vi "IVI DC Power Supply RT Driver VI.vi"(6 "Device Clock":string, 9 "Device Inputs FIFO":refnum<k33>, 10 "Device Outputs FIFO":refnum<k33>, 11 "Device Reference":T1 format="%.0x") -> ()   [LabVIEW 2011, in "IVI DC Power Supply Custom Device.lvlib"]
uses:
  IVI DC Power Supply Custom Device.lvlib
  <vilib>/NI Veristand/Custom Device API/Custom Device Item Ref.ctl
  <vilib>/NI Veristand/Custom Device API/Custom Device Channel Type.ctl
  <vilib>/Platform/TimedLoop/XDataNode/timing_clust.ctl
  <vilib>/Platform/TimedLoop/XDataNode/nitl_modes.ctl
  <vilib>/Platform/TimedLoop/XDataNode/wakeup.ctl
  Global.vi
  <vilib>/NI Veristand/Custom Device API/Get Item Property (Double).vi
  <vilib>/Platform/TimedLoop/XDataNode/XDataNode.xnode
  <vilib>/Platform/TimedLoop/XDataNode/XDNodeRunTimeDep.lvlib
  <vilib>/NI Veristand/Custom Device API/Custom Device API.lvlib
  <vilib>/NI Veristand/Custom Device Tools/Custom Device Utility Library/Custom Device Utility Library.lvlib
panel:
  in  "Status Notifier":refnum<notifier>
  # "Custom Device Template\nv1.0"
  # "Use this template as a starting point for creating a custom device code module. The input controls shown here are specially named controls that the system will use to provide the device loop with data. The controls are not required for the device loop to run. For instance, if the device doesn't produce any output data, then you don't need the Device Outputs FIFO control. If you do use these controls, however, they need to have these exact names to be functional."
  # "The optional status notifier element is used to notify the RT engine of the last state of the custom device, and to indicate the device has completed execution. If this control is not used, a default No Error value is returned to the system when the device finishes execution.\n\nNote: This error state is not checked until the system shuts down. Use an output status channel to send more immediate status values to the system."
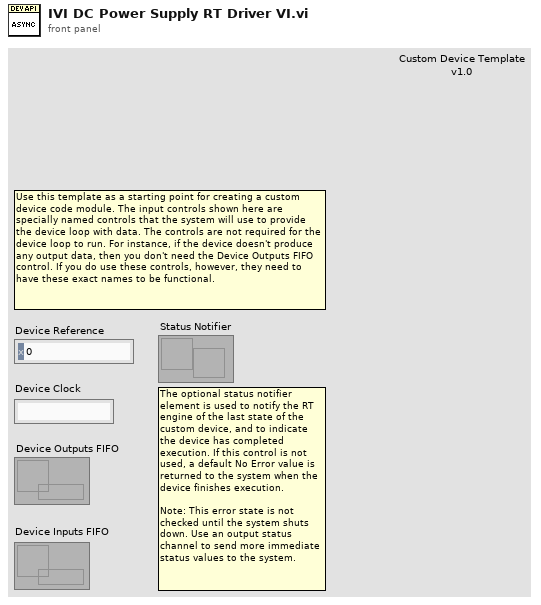
[diagram p1: front panel]
types:
  T1 = typedef "Custom Device API.lvlib/Custom Device Item Ref.ctl" = u64
  T2 = typedef "Custom Device API.lvlib/Custom Device Channel Type.ctl" = enum16{"Input", "Output"}
  T3 = typedef "Custom Device API.lvlib/Custom Device Timed Loop Priority.ctl" = enum32{"Low", "Medium", "High"}
  T4 = typedef "XDNodeRunTimeDep.lvlib/timing_clust.ctl" = cluster{"Expected End [f-1]":u64, "Actual End [f-1]":u64, "Finished Late? [f-1]":bool, "Expected End [i-1]":u64, "Actual End [i-1]":u64, "Finished Late? [i-1]":bool, "Expected Start [i]":u64, "Actual Start [i]":u64, "Expected Start [f]":u64, "Actual Start [f]":u64, "Source Name":string, "Structure Name":string, "Period":i64, "Deadline":i64, "Offset":i64, "Start":i64, "Priority":i32, "Timeout":i32, "Mode":T5, "Wakeup Reason":T6, "Error":errorcluster, "Source Type":string, "Secondary Source Type":string, "Global End Time":u64, "Global Start Time":u64, "Frame Duration":u64, "Iteration Duration":u64, "Assigned CPU":i32, "I/O Scan Engine Mode":u32}
  T5 = typedef "XDNodeRunTimeDep.lvlib/nitl_modes.ctl" = enum32{"No Change", "Process missed periods, maintain original phase", "Discard missed periods, maintain original phase", "Process missed periods, ignore original phase", "Discard missed periods, ignore original phase"}
  T6 = typedef "XDNodeRunTimeDep.lvlib/wakeup.ctl" = enum32{"Normal", "Aborted", "Asynchronous wakeup", "Timing source error", "Timed loop error", "Timeout"}
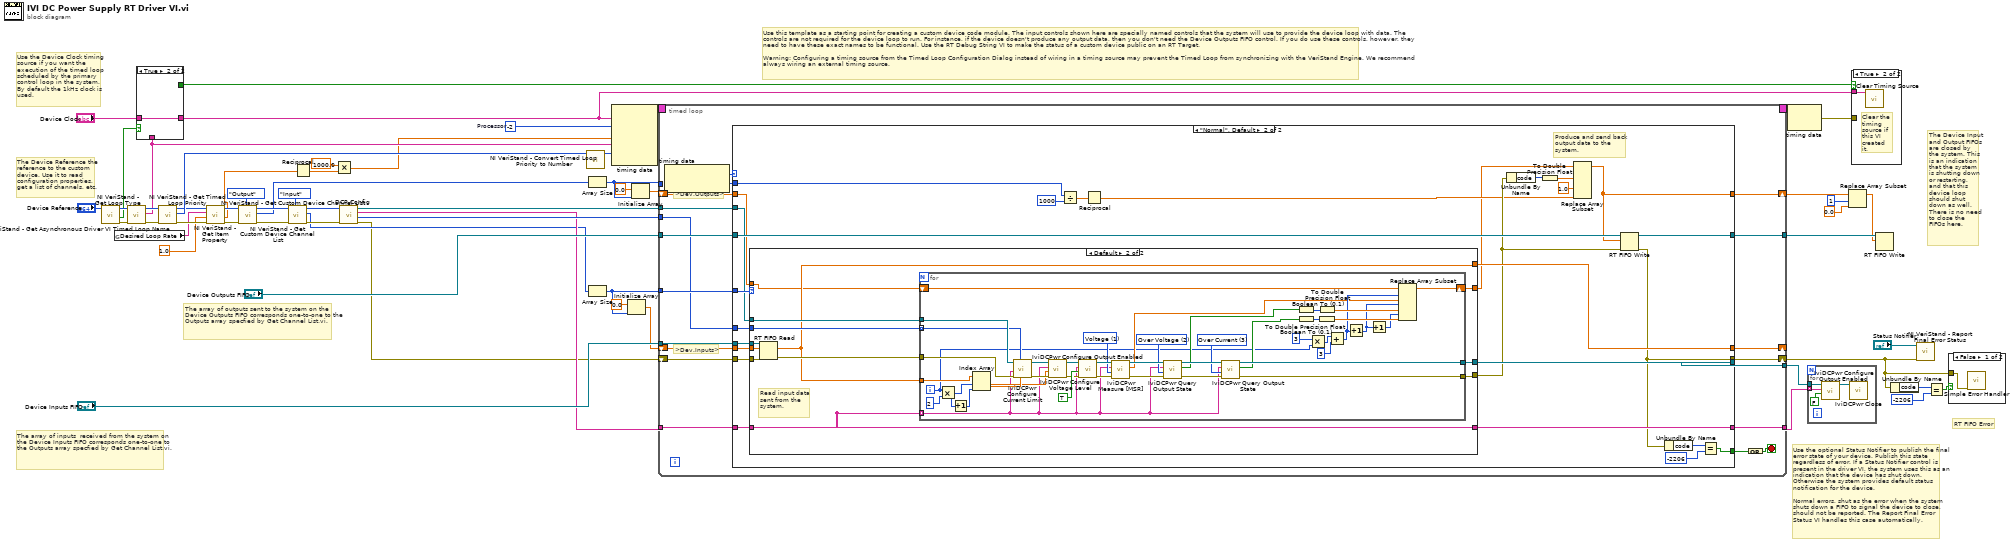
[diagram p0: block diagram]
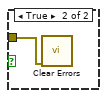
[diagram p2: hidden frame]
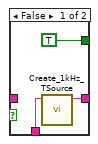
[diagram p4: hidden frame]
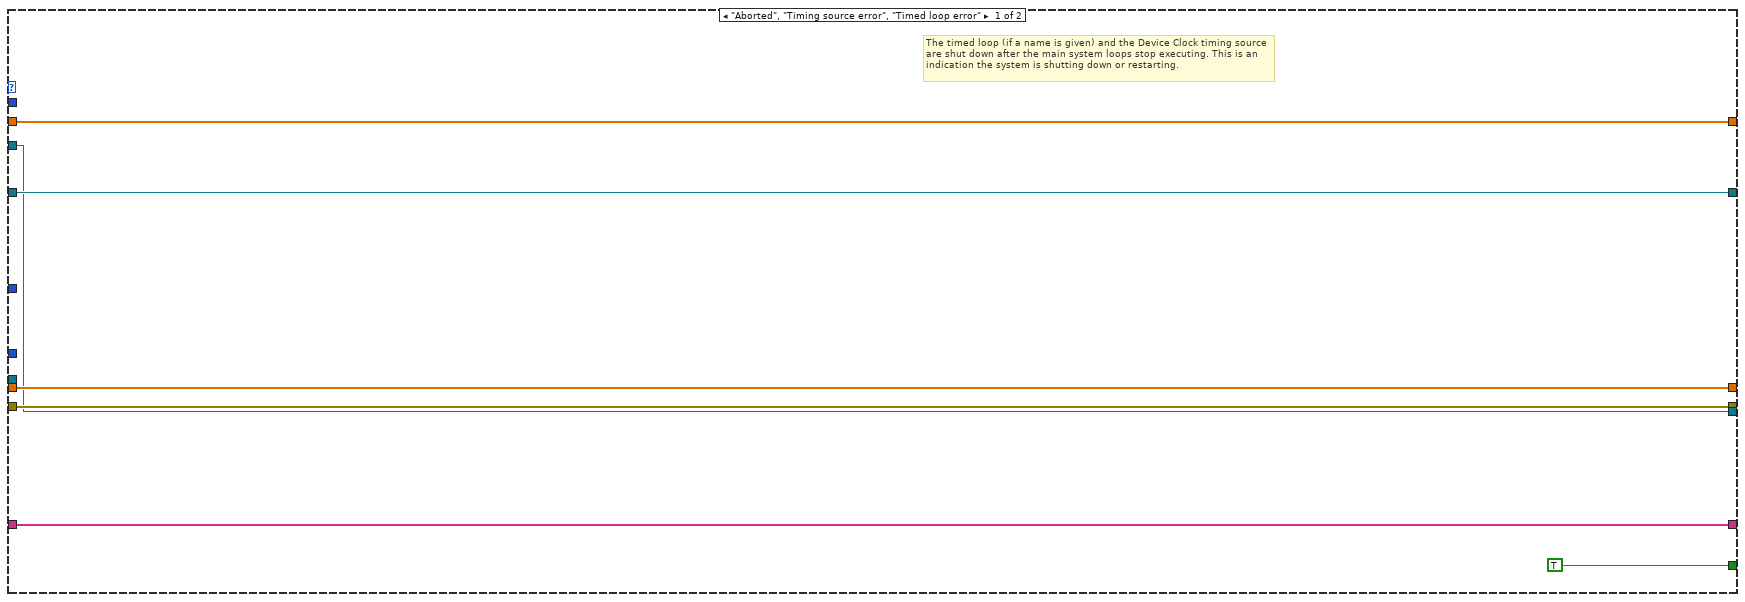
[diagram p5: hidden frame]
diagram:
  w41 = -2  # Processor
  # "RT FIFO Error"
  # "The array of inputs  received from the system on the Device Inputs FIFO corresponds one-to-one to the Outputs array specfied by Get Channel List.vi."
  # "Use the optional Status Notifier to publish the final error state of your device. Publish this state regardless of error. If a Status Notifier control is present in the driver VI, the system uses this as an indication that the device has shut down. Otherwise the system provides default status notification for the device.\n\nNormal errors, shut as the error when the system shuts down a FIFO to signal the device to close, should not be reported. The Report Final Error Status VI handles this case automatically."
  # "The Device Input and Output FIFOs are closed by the system. This is an indication that the system is shutting down or restarting, and that this device loop should shut down as well. There is no need to close the FIFOs here."
  # "The array of outputs sent to the system on the Device Outputs FIFO corresponds one-to-one to the Outputs array specfied by Get Channel List.vi."
  # "The Device Reference the reference to the custom device. Use it to read configuration properties, get a list of channels, etc."
  # "Use the Device Clock timing source if you want the execution of the timed loop scheduled by the primary control loop in the system. \nBy default the 1kHz clock is used."
  # "Use this template as a starting point for creating a custom device code module. The input controls shown here are specially named controls that the system will use to provide the device loop with data. The controls are not required for the device loop to run. For instance, if the device doesn't produce any output data, then you don't need the Device Outputs FIFO control. If you do use these controls, however, they need to have these exact names to be functional. Use the RT Debug String VI to make the status of a custom device public on an RT Target.\n\nWarning: Configuring a timing source from the Timed Loop Configuration Dialog instead of wiring in a timing source may prevent the Timed Loop from synchronizing with the VeriStand Engine. We recommend always wiring an external timing source."
  n1 = call <vilib>:"NI VeriStand - Get Loop Type.vi"("Device Ref in"="Device Reference") -> ("error out"=w39:errorcluster, "Use Device Clock"=w36:bool, "Device Ref out"=w38:T1)  [unwired: 1 in, 7 out]
  n2 = global read "Global.vi" "Desired Loop Rate"() -> (w10:string)
  n3 = call <vilib>:"NI VeriStand - Get Asynchronous Driver VI Timed Loop Name.vi"("error in (no error)"=w39, "Device Ref in"=w38) -> ("error out"=w44:errorcluster, "Device Timed Loop Name"=w30:string, "Device Ref out"=w58:T1)  [unwired: 7 out]
  n4 = case shown="True" w36 {
    tunnel: "Device Clock" -> [_ w62]
    tunnel: [w61 w62] -> w31
    tunnel: [TRUE _] -> w32
    tunnel: w30 -> [w59 _]
    frame False {
      n5 = call <vilib>:"Create_1kHz_TSource.vi"("name (in)"=w59) -> ("name (out)"=w61:string)  [unwired: 1 in, 9 out]
    }
    frame True {
    }
  }
  n6 = call <vilib>:"NI VeriStand - Get Timed Loop Priority.vi"("error in (no error)"=w44, "Device Ref in"=w58) -> ("error out"=w14:errorcluster, "Priority"=w43:T3, "Device Ref out"=w11:T1)  [unwired: 7 out]
  n7 = call-poly <vilib>:"NI VeriStand - Get Item Property.vi"("error in (no error)"=w14, "Default Value"=1.0, "Property Name"=w10, "Item Ref in"=w11) -> ("error out"=w13:errorcluster, "Value"=w7:dbl, "Item Ref out"=w12:T1)  [unwired: 4 in, 1 out]
  n8 = call <vilib>:"NI VeriStand - Get Custom Device Channel List.vi"("Channel Type"=Custom_Device_Channel_Type."Output", "error in (no error)"=w13, "Device Ref in"=w12) -> ("error out"=w47:errorcluster, "Specified Channel Ref List"=w28:T1[], "Device Ref out"=w48:T1)  [unwired: 6 out]
  n9 = call <vilib>:"NI VeriStand - Get Custom Device Channel List.vi"("Channel Type"=Custom_Device_Channel_Type."Input", "error in (no error)"=w47, "Device Ref in"=w48) -> ("error out"=w29:errorcluster, "Specified Channel Ref List"=w16:T1[], "Device Ref out"=w22:T1)  [unwired: 6 out]
  n10 = Reciprocal(x=w7) -> (1/x=w8:dbl)
  n11 = Multiply(x=1000.0, y=w8) -> (x*y=w5:dbl)
  n12 = call "DCP Config.vi"("error in (no error)"=w29, "Device Reference In"=w22) -> ("error out"=w15:errorcluster, "Limit Behaviour"=w18:u16[], "Channels"=w17:string[], "instrument handle out"=w19:refnum<k15>)  [unwired: 6 in]
  n13 = call <vilib>:"NI VeriStand - Convert Timed Loop Priority to Number.vi"("Priority"=w43) -> ("Numeric Priority"=w42:i32)  [unwired: 10 out]
  n14 = Array Size(array=w28) -> (size(s)=w45:i32)
  n15 = Array Size(array=w16) -> (size(s)=w40:i32)
  n16 = node-c288(w31, w41, w5, w30, w42) -> (w55:T4)
  n17 = Initialize Array(0.0 ("element"), w40) -> (w50:dbl[])
  n18 = Initialize Array(0.0 ("element"), w45) -> (w51:dbl[])
  n19 = timed-loop {
    timing: w55 -> [_]
    timing-out: [_] -> w54
    shift-right: [w80] -> _
    shift-left: w50 -> [w81]
    shift-right: [w78] -> w27
    shift-left: w51 -> [w79]
    tunnel: w45 -> [_]
    tunnel: "Device Outputs FIFO" -> [w77]
    tunnel: "Device Inputs FIFO" -> [w76]
    tunnel: w40 -> [w73]
    tunnel: w19 -> [w72]
    tunnel: [w71] -> w24
    tunnel: [w70] -> w21
    tunnel: w17 -> [w68]
    tunnel: [w69] -> w20
    tunnel: w18 -> [w67]
    shift-right: [w63] -> w1
    shift-left: w15 -> [w65]
    stop <- w74 stop-if-true
    # ">Dev.Outputs>"
    # ">Dev.Inputs>"
    n20 = node-c288() -> (w64:T6, w66:i64)  [unwired: 1 out]
    n21 = case shown="\"Normal\", Default" w64 {
      tunnel: w65 -> [w87 w112]
      tunnel: w81 -> [w88 w113]
      tunnel: [w87 w89] -> w63
      tunnel: [w88 w110] -> w80
      tunnel: w79 -> [w86 w94]
      tunnel: [w86 w95] -> w78
      tunnel: w77 -> [w84 w115]
      tunnel: w76 -> [_ w114]
      tunnel: [TRUE w90] -> w75
      tunnel: w73 -> [_ w111]
      tunnel: w72 -> [w83 w105]
      tunnel: [w84 w107] -> w71
      tunnel: [w83 w104] -> w70
      tunnel: w68 -> [w82 w102]
      tunnel: [w82 w103] -> w69
      tunnel: w67 -> [_ w101]
      tunnel: w66 -> [_ w97]
      frame "Aborted", "Timing source error", "Timed loop error" {
        # "The timed loop (if a name is given) and the Device Clock timing source are shut down after the main system loops stop executing. This is an indication the system is shutting down or restarting."
      }
      frame "Normal", Default {
        # "Produce and send back output data to the system."
        n22 = case shown="Default" w111 {
          tunnel: w114 -> [_ w132]
          tunnel: w113 -> [w120 w131]
          tunnel: [w120 w123] -> w110
          tunnel: [w119 w127] -> w100
          tunnel: w112 -> [w119 w130]
          tunnel: w105 -> [w118 w129]
          tunnel: [w118 w126] -> w104
          tunnel: [w117 w125] -> w103
          tunnel: w102 -> [w117 w125]
          tunnel: w101 -> [_ w124]
          tunnel: w94 -> [w116 w122]
          tunnel: [w116 w121] -> w93
          frame 0 {
            # "No inputs to read\nfrom system. Inputs FIFO not created in this case, so don't write to it."
          }
          frame Default {
            # "Read input data sent from the system."
            n23 = RT FIFO Read(0:w132, 1:w131, 3:w130) -> (9:w123:dbl[], 11:w128:errorcluster)  [unwired: 4 out]
            n24 = for {
              tunnel: w129 -> [w169]
              tunnel: w128 -> [w168]
              tunnel: [w156] -> w127
              tunnel: [w155] -> w126
              tunnel: w125 -> [w154] mode=indexing
              tunnel: w123 -> [w152]
              tunnel: w124 -> [w153] mode=indexing
              shift-right: [w134] -> w121
              shift-left: w122 -> [w135]
              i -> [w133]
              w157 = 3 items=["Constant Voltage"=0, "Constant Current"=1, "Unregulated"=4, "Over Voltage"=2, "Over Current"=3] ("output state (Constant Voltage)")
              w158 = 2 items=["Constant Voltage"=0, "Constant Current"=1, "Unregulated"=4, "Over Voltage"=2, "Over Current"=3] ("output state (Constant Voltage)")
              w159 = 1 items=["Voltage"=1, "Current"=0] ("measurement type (voltage)")
              n25 = Multiply(x=w133, y=2) -> (x*y=w151:i32)
              n26 = Increment(x=w151) -> (x+1=w150:i32)
              n27 = Index Array(array=w152, index #1=w151, index #2=w150) -> (element #1=w166:dbl, element #2=w167:dbl)
              n28 = call <vilib>:"IviDCPwr Configure Current Limit.vi"("limit (0.0 Amps)"=w167, "behavior (regulate)"=w153, "error in (no error)"=w168, "channel name (\"CHANNEL1\")"=w154, "instrument handle"=w169) -> ("error out"=w170:errorcluster, "instrument handle out"=w171:refnum<k15>)  [unwired: 5 in]
              n29 = call <vilib>:"IviDCPwr Configure Voltage Level.vi"("error in (no error)"=w170, "level (0.0 Volts)"=w166, "channel name (\"CHANNEL1\")"=w154, "instrument handle"=w171) -> ("error out"=w172:errorcluster, "instrument handle out"=w173:refnum<k15>)  [unwired: 6 in]
              n30 = call <vilib>:"IviDCPwr Configure Output Enabled.vi"("error in (no error)"=w172, "enabled (true)"=TRUE, "channel name (\"CHANNEL1\")"=w154, "instrument handle"=w173) -> ("error out"=w161:errorcluster, "instrument handle out"=w160:refnum<k15>)  [unwired: 6 in]
              n31 = call <vilib>:"IviDCPwr Measure [MSR].vi"("error in (no error)"=w161, "measurement type (voltage)"=w159, "channel name (\"CHANNEL1\")"=w154, "instrument handle"=w160) -> ("error out"=w163:errorcluster, "measurement"=w136:dbl, "instrument handle out"=w162:refnum<k15>)  [unwired: 5 out]
              n32 = call <vilib>:"IviDCPwr Query Output State.vi"("error in (no error)"=w163, "output state (Constant Voltage)"=w158, "channel name (\"CHANNEL1\")"=w154, "instrument handle"=w162) -> ("error out"=w164:errorcluster, "in state"=w137:bool, "instrument handle out"=w165:refnum<k15>)  [unwired: 5 out]
              n33 = call <vilib>:"IviDCPwr Query Output State.vi"("error in (no error)"=w164, "output state (Constant Voltage)"=w157, "channel name (\"CHANNEL1\")"=w154, "instrument handle"=w165) -> ("error out"=w156:errorcluster, "in state"=w138:bool, "instrument handle out"=w155:refnum<k15>)  [unwired: 5 out]
              n34 = Boolean To (0,1)(Boolean=w138) -> (0, 1=w139:i16)
              n35 = Boolean To (0,1)(Boolean=w137) -> (0, 1=w140:i16)
              n36 = Multiply(x=3, y=w133) -> (x*y=w146:i32)
              n37 = To Double Precision Float(number=w139) -> (double precision float=w147:dbl)
              n38 = To Double Precision Float(number=w140) -> (double precision float=w148:dbl)
              n39 = Add(x=w146, y=3 ("x")) -> (x+y=w144:i32)
              n40 = Increment(x=w144) -> (x+1=w142:i32)
              n41 = Increment(x=w142) -> (x+1=w143:i32)
              n42 = Replace Array Subset(array=w135, new element #1=w136, index #1=w144, new element #2=w148, index #2=w142, new element #3=w147, index #3=w143) -> (w134:dbl[])
            }
          }
        }
        n43 = Divide(x=w97, y=i64 1000) -> (x/y=w98:dbl)
        n44 = Reciprocal(x=w98) -> (1/x=w99:dbl)
        n45 = Unbundle By Name(w100) -> ("code"=w106:i32)
        n46 = To Double Precision Float(number=w106) -> (double precision float=w108:dbl)
        n47 = Replace Array Subset(array=w93, new element #1=w108, new element #2=1.0 ("new element/subarray"), new element #3=w99) -> (w95:dbl[])  [unwired: 3 in]
        n48 = RT FIFO Write(0:w115, 1:w95, 3:w100) -> (8:w107:refnum<k33>, 11:w89:errorcluster)  [unwired: 1 in, 3 out]
        n49 = Unbundle By Name(w89) -> ("code"=w91:i32)
        n50 = Equal?(x=w91, y=-2206) -> (x = y?=w90:bool)
      }
    }
    n51 = Compound Arithmetic op=OR(w75) -> (w74:bool)
  }
  n52 = node-c288(w54) -> (w33:errorcluster)
  n53 = for {
    tunnel: w21 -> [w182]
    tunnel: w20 -> [w180] mode=indexing
    n54 = call <vilib>:"IviDCPwr Configure Output Enabled.vi"("enabled (true)"=FALSE, "channel name (\"CHANNEL1\")"=w180, "instrument handle"=w182) -> ("instrument handle out"=w181:refnum<k15>)  [unwired: 7 in, 1 out]
    n55 = call <vilib>:"IviDCPwr Close.vi"("instrument handle"=w181) -> ()  [unwired: 10 in, 1 out]
  }
  n56 = Replace Array Subset(array=w27, new element=0.0 ("new element/subarray"), index=1) -> (w23:dbl[])
  n57 = case shown="True" w32 {
    tunnel: w33 -> [_ _]
    tunnel: w31 -> [_ w183]
    frame False {
    }
    frame True {
      # "Clear the timing source if this VI created it."
      n58 = call <vilib>:"Clear Timing Source.vi"("name"=w183) -> ()  [unwired: 1 in, 10 out]
    }
  }
  n59 = RT FIFO Write(0:w24, 1:w23) -> ()  [unwired: 2 in, 5 out]
  n60 = Unbundle By Name(w1) -> ("code"=w4:i32)
  n61 = call <vilib>:"NI VeriStand - Report Final Error Status.vi"("error in (no error)"=w1, "Status Notifier"="Status Notifier") -> ()  [unwired: 1 in, 9 out]
  n62 = Equal?(x=w4, y=-2206) -> (x = y?=w2:bool)
  n63 = case shown="False" w2 {
    tunnel: w1 -> [w184 w185]
    frame False {
      n64 = call <vilib>:"Simple Error Handler.vi"("error in (no error)"=w184) -> ()  [unwired: 4 in, 5 out]
    }
    frame True {
      n65 = call <vilib>:"Clear Errors.vi"("error in (no error)"=w185) -> ()  [unwired: 6 in, 1 out]
    }
  }
